vi "edit_component_sequence_dialog.vi"(1 "show configuration?":bool=TRUE, 2 "default folder path":path, 3 "show label?":bool=TRUE, 5 "component specification list in":T1[](array[typedef]), 9 "default":string, 11 "error in (no error)":errorcluster, 12 "choose default?":bool=TRUE, 14 "show settings?":bool=TRUE) -> (6 "component specification list out":T1[](array[typedef]), 10 "default":string, 15 "error out":errorcluster)   [LabVIEW 2010, in "GenericComponent.lvclass"]
uses:
  GenericComponent.lvclass
  clusters/plugin_specification.ctl
  <vilib>/Utility/miscctls.llb/LVPointTypeDef.ctl
panel:
  in  "set_preselected_default":bool=TRUE
  in  "preselected default":string(combo)
  in  "down button":bool
  in  "up button":bool
  in  "cancel button":bool
  in  "edit button":bool
  in  "delete button":bool
  in  "done button":bool
  in  "add button":bool
  in  "Plug-ins":i32(listbox)
  # "Edit component sequence"
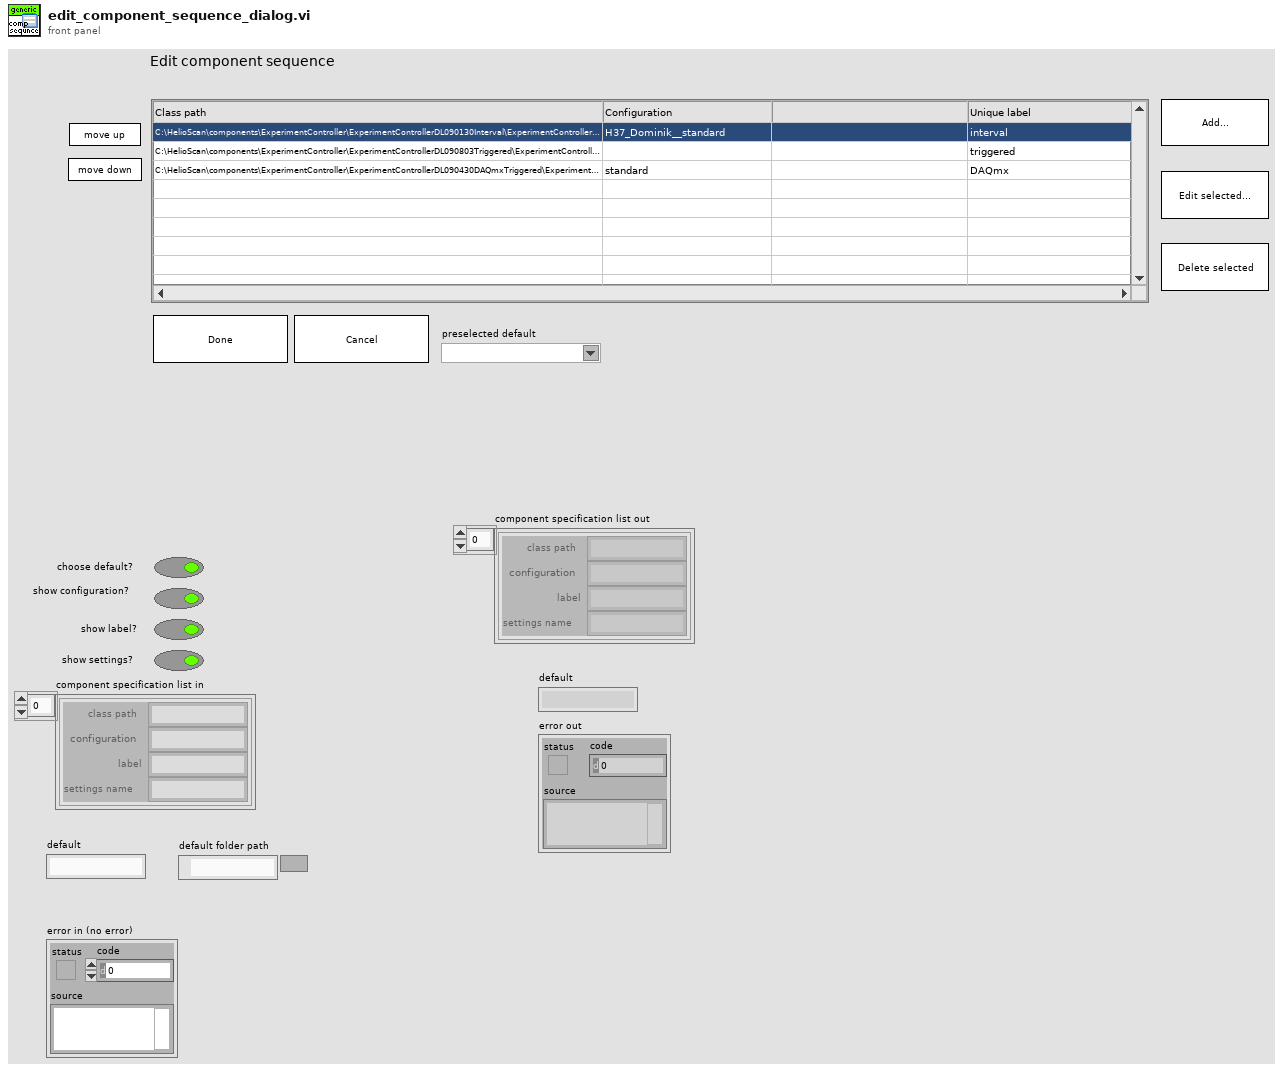
[diagram p1: front panel]
types:
  T1 = typedef "plugin_specification.ctl" = cluster{"class path":string, "configuration":string, "label":string, "settings name":string}
  T2 = typedef "LVPointTypeDef.ctl" = cluster{"Horizontal":i16, "Vertical":i16}
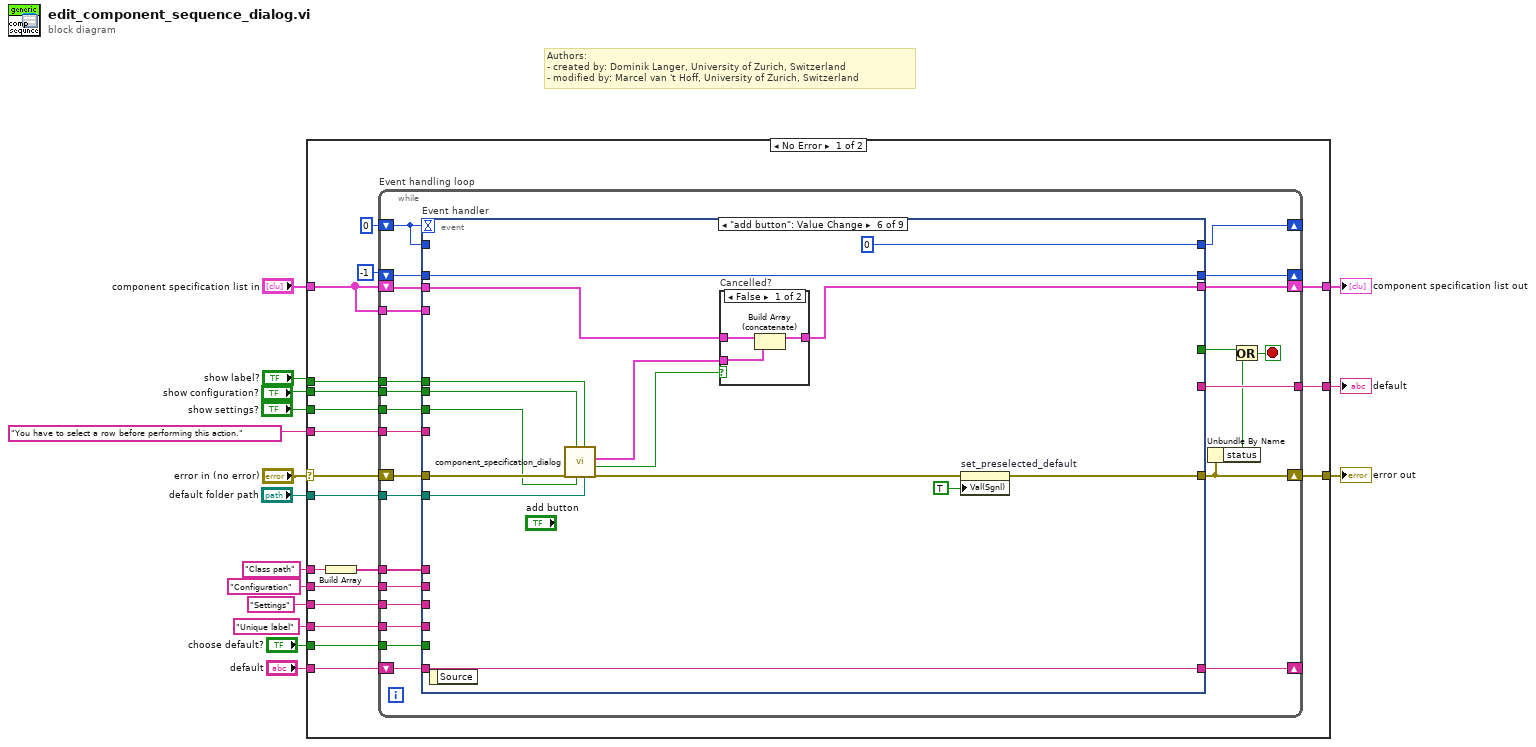
[diagram p0: block diagram]
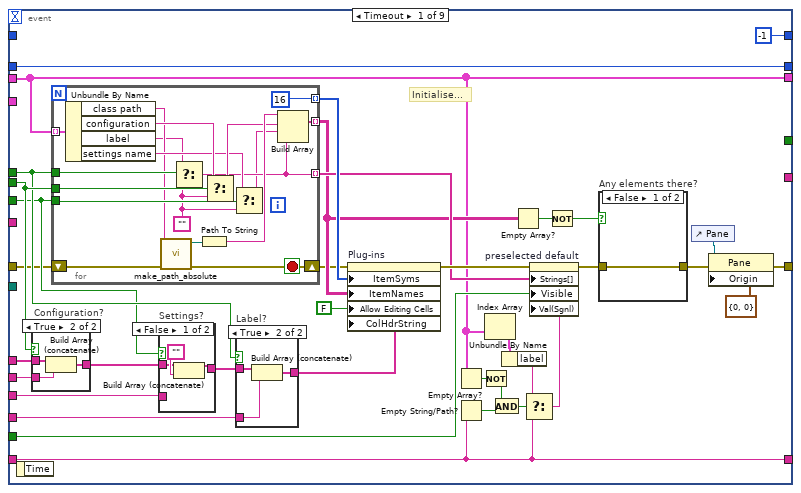
[diagram p2: hidden frame]
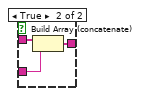
[diagram p3: hidden frame]
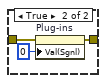
[diagram p4: hidden frame]
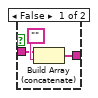
[diagram p5: hidden frame]
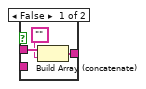
[diagram p6: hidden frame]
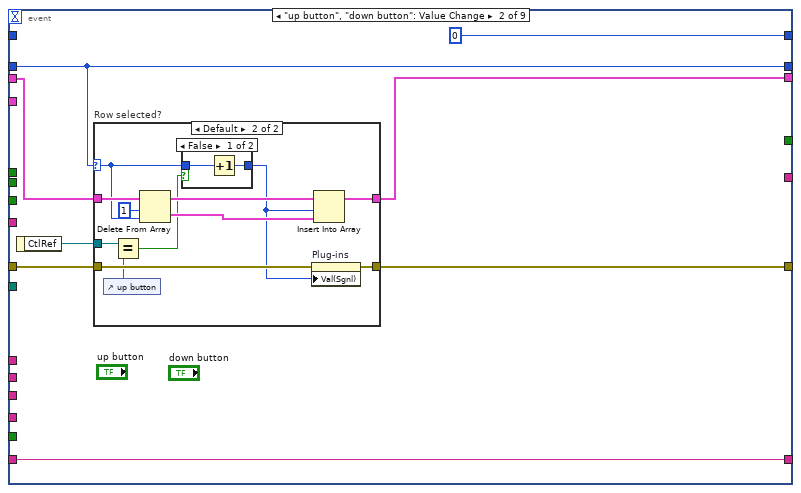
[diagram p7: hidden frame]
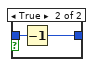
[diagram p9: hidden frame]
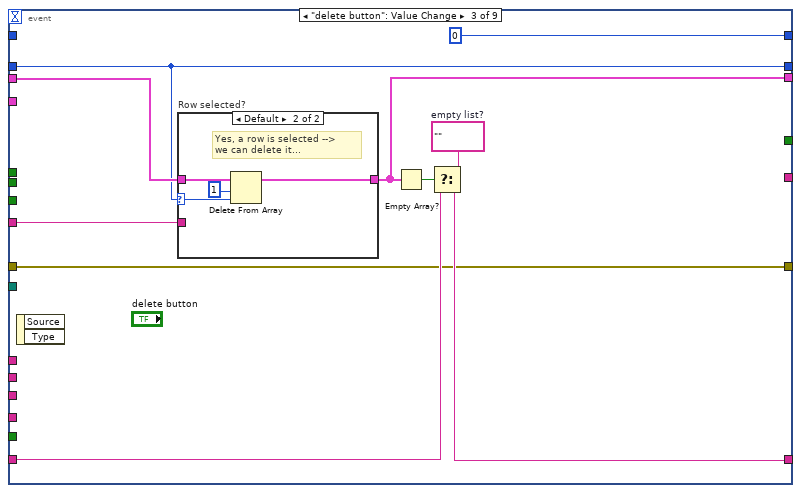
[diagram p10: hidden frame]
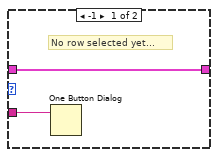
[diagram p11: hidden frame]
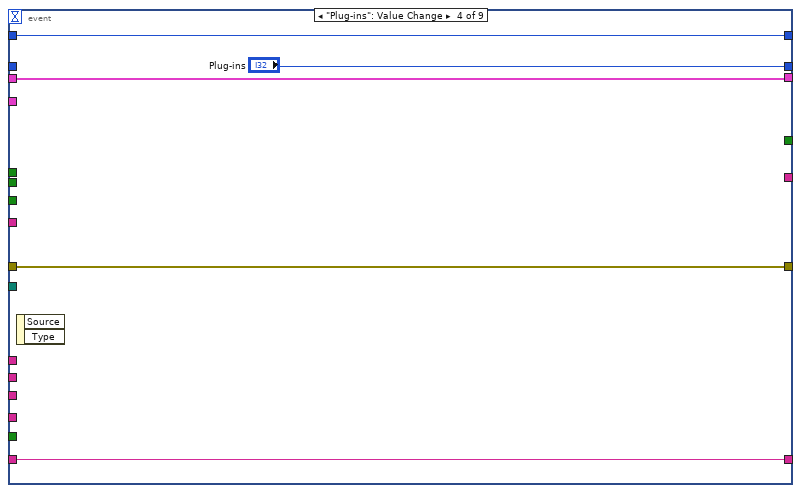
[diagram p12: hidden frame]
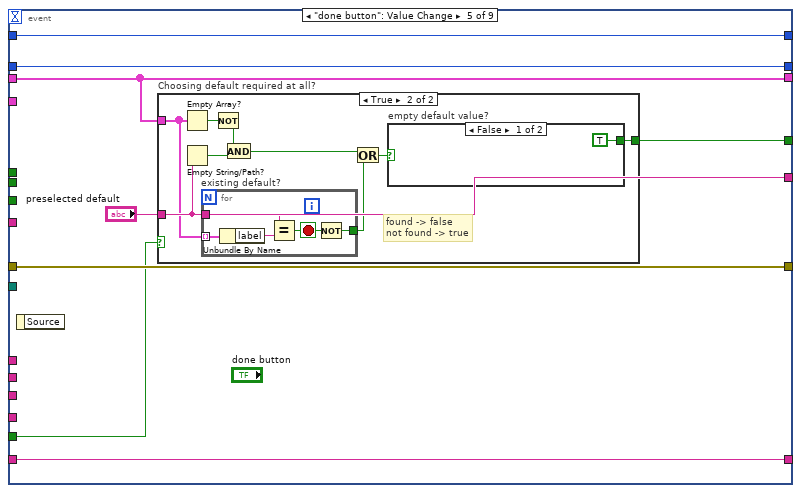
[diagram p13: hidden frame]
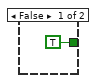
[diagram p14: hidden frame]
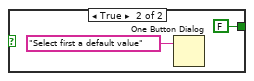
[diagram p15: hidden frame]
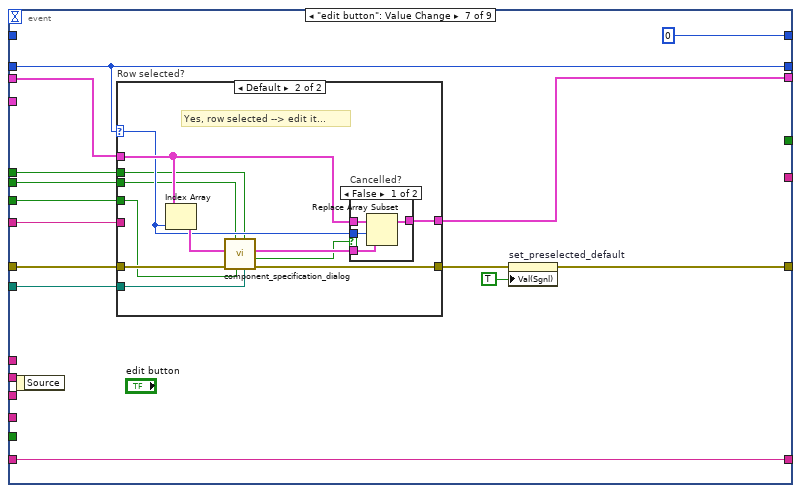
[diagram p17: hidden frame]
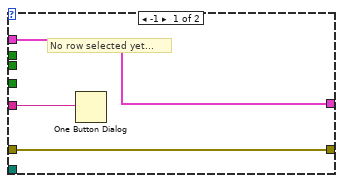
[diagram p18: hidden frame]
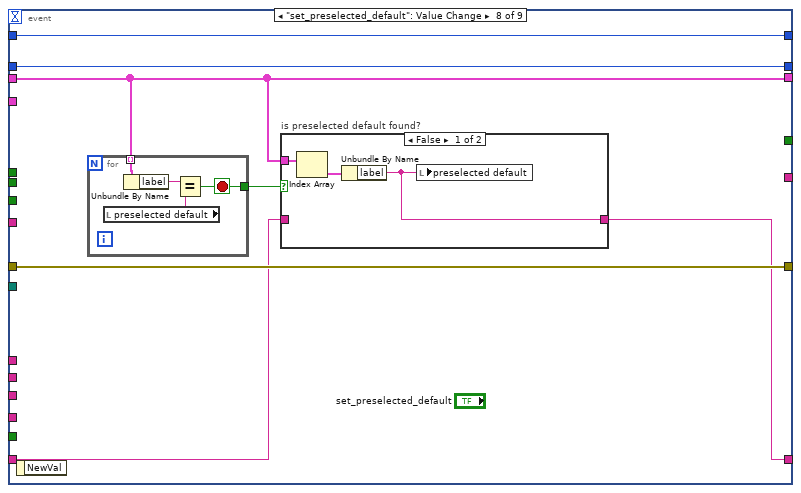
[diagram p20: hidden frame]
diagram:
  # "Authors: \n- created by: Dominik Langer, University of Zurich, Switzerland\n- modified by: Marcel van 't Hoff, University of Zurich, Switzerland"
  n1 = case shown="No Error" "error in (no error)" {
    selector: "error in (no error)" -> [w35 w284]
    tunnel: [w34 w284] -> w15
    tunnel: "component specification list in" -> [w31 _]
    tunnel: "You have to select a row before performing this action." -> [w30 _]
    tunnel: [w29 _] -> w12
    tunnel: "show configuration?" -> [w28 _]
    tunnel: "show label?" -> [w27 _]
    tunnel: "Class path" -> [w26 _]
    tunnel: "Configuration" -> [w23 _]
    tunnel: "Unique label" -> [w24 _]
    tunnel: "choose default?" -> [w22 _]
    tunnel: [w21 _] -> w5
    tunnel: "default" -> [w20 _]
    tunnel: "show settings?" -> [w19 _]
    tunnel: "Settings" -> [w18 _]
    tunnel: "default folder path" -> [w17 _]
    frame No Error {
      n2 = Build Array(w26) -> (w25:string[])
      n3 = while "Event handling loop" {
        shift-right: [w40] -> w34
        shift-left: w35 -> [w60]
        shift-right: [w58] -> _
        shift-left: 0 -> [w59]
        shift-right: [w56] -> w29
        shift-left: w31 -> [w57]
        shift-right: [w54] -> _
        shift-left: -1 -> [w55]
        tunnel: w31 -> [w53]
        tunnel: w30 -> [w52]
        tunnel: w28 -> [w51]
        tunnel: w27 -> [w50]
        tunnel: w25 -> [w49]
        tunnel: w23 -> [w48]
        tunnel: w24 -> [w47]
        tunnel: w22 -> [w46]
        tunnel: [w45] -> w21
        tunnel: w19 -> [w43]
        tunnel: w18 -> [w42]
        tunnel: w17 -> [w41]
        shift-right: [w36] -> _
        shift-left: w20 -> [w44]
        stop <- w37 stop-if-true
        n4 = event "Event handler" shown="[5] \"add button\": Value Change" {
          selector: _ -> [_ _ _ _ _ _ _ _ _]
          dyn-events: _ -> [_ _ _ _ _ _ _ _ _]
          timeout: w59 -> [_ _ _ _ _ _ _ _ _]
          tunnel: w60 -> [w75 w141 w163 w182 w190 w224 w242 w267 w282]
          tunnel: w59 -> [_ _ _ w183 w191 _ _ w269 w283]
          tunnel: [-1 0 0 w183 w191 0 0 w269 w283] -> w58
          tunnel: [w63 w140 w163 w182 w190 w212 w230 w267 w282] -> w40
          tunnel: w57 -> [w69 w143 w172 w181 w187 w219 w241 w264 _]
          tunnel: [_ _ _ _ w185 _ _ _ TRUE] -> w38
          tunnel: [w69 w142 w168 w181 w187 w222 w240 w264 w279] -> w56
          tunnel: w55 -> [w93 w139 w170 _ w189 w220 w238 w268 w281]
          tunnel: [w93 w139 w170 "Plug-ins" w189 w220 w238 w268 w281] -> w54
          tunnel: w53 -> [_ _ _ _ _ _ _ _ w279]
          tunnel: w52 -> [_ _ w169 _ _ _ w237 _ _]
          tunnel: w51 -> [w90 _ _ _ _ w216 w236 _ _]
          tunnel: w50 -> [w89 _ _ _ _ w217 w235 _ _]
          tunnel: w49 -> [w92 _ _ _ _ _ _ _ _]
          tunnel: w48 -> [w91 _ _ _ _ _ _ _ _]
          tunnel: w47 -> [w78 _ _ _ _ _ _ _ _]
          tunnel: w46 -> [w86 _ _ _ w184 _ _ _ _]
          tunnel: [_ _ _ _ "preselected default" _ _ _ w278] -> w45
          tunnel: w44 -> [w61 w137 w165 w179 w188 w210 w229 w266 w278]
          tunnel: w43 -> [w76 _ _ _ _ w215 w234 _ _]
          tunnel: w42 -> [w79 _ _ _ _ _ _ _ _]
          tunnel: w41 -> [_ _ _ _ _ w214 w233 _ _]
          tunnel: [w61 w137 w164 w179 w188 w210 w229 w265 w278] -> w36
          event Timeout {
            # "Initialise..."
            n5 = event-data() -> ()  [unwired: 2 out]
            n6 = case "Configuration?" shown="True" w90 {
              tunnel: w92 -> [w115 w118]
              tunnel: w91 -> [_ w117]
              tunnel: [w114 w116] -> w81
              frame False {
                n7 = Build Array (concatenate)(w115, "") -> (w114:string[])
              }
              frame True {
                n8 = Build Array (concatenate)(w118, w117) -> (w116:string[])
              }
            }
            n9 = for {
              tunnel: w69 -> [w136] mode=indexing
              tunnel: [w134] -> w82 mode=indexing
              tunnel: [16] -> w94 mode=indexing
              tunnel: w89 -> [w132]
              tunnel: w90 -> [w131]
              tunnel: [w125] -> w87 mode=indexing
              tunnel: w76 -> [w128]
              shift-right: [w119] -> w74
              shift-left: w75 -> [w123]
              stop <- w119 stop-if-true
              w126 = ""
              n10 = Unbundle By Name(w136) -> ("class path"=w122:string, "configuration"=w130:string, "label"=w120:string, "settings name"=w127:string)
              n11 = call "make_path_absolute.vi"("error in (no error)"=w123, "relative path"=w122) -> ("error out"=w119:errorcluster, "absolute path"=w121:path)  [unwired: 8 in]
              n12 = Select(t=w120, s=w132, f=w126) -> (s? t:f=w125:string)
              n13 = Path To String(path=w121) -> (string=w135:string)
              n14 = Select(t=w130, s=w131, f=w126) -> (s? t:f=w129:string)
              n15 = Select(t=w127, s=w128, f=w126) -> (s? t:f=w124:string)
              n16 = Build Array(w135, w129, w124, w125) -> (w134:string[])
            }
            n17 = case "Settings?" shown="False" w76 {
              tunnel: w81 -> [w98 w102]
              tunnel: w79 -> [_ w101]
              tunnel: [w97 w100] -> w80
              frame False {
                n18 = Build Array (concatenate)(w98, "") -> (w97:string[])
              }
              frame True {
                n19 = Build Array (concatenate)(w102, w101) -> (w100:string[])
              }
            }
            n20 = case "Label?" shown="True" w89 {
              tunnel: w80 -> [w107 w112]
              tunnel: w78 -> [_ w111]
              tunnel: [w108 w110] -> w77
              frame False {
                n21 = Build Array (concatenate)(w107, "") -> (w108:string[])
              }
              frame True {
                n22 = Build Array (concatenate)(w112, w111) -> (w110:string[])
              }
            }
            n23 = property on="Plug-ins" class="MCListbox (strict)"(error in=w74, "ItemSyms"=w94, "ItemNames"=w82, "Allow Editing Cells"=FALSE, "ColHdrString"=w77) -> (error out=w88:errorcluster)  [unwired: 1 in, 1 out]
            n24 = Empty Array?(array=w69) -> (empty?=w73:bool)
            n25 = Empty String/Path?(string/path=w61) -> (empty?=w71:bool)
            n26 = Not(x=w73) -> (.not. x?=w72:bool)
            n27 = Index Array(array=w69) -> (element=w70:T1)  [unwired: 1 in]
            n28 = And(x=w72, y=w71) -> (x .and. y?=w67:bool)
            n29 = Unbundle By Name(w70) -> ("label"=w68:string)
            n30 = Empty Array?(array=w82) -> (empty?=w84:bool)
            n31 = Select(t=w68, s=w67, f=w61) -> (s? t:f=w66:string)
            n32 = property on="preselected default" class="CmbBox"(error in=w88, "Strings[]"=w87, "Visible"=w86, "Val(Sgnl)"=w66) -> (error out=w85:errorcluster)  [unwired: 1 in, 1 out]
            n33 = Not(x=w84) -> (.not. x?=w83:bool)
            n34 = case "Any elements there?" shown="False" w83 {
              tunnel: w85 -> [w103 w106]
              tunnel: [w103 w105] -> w62
              frame False {
              }
              frame True {
                n35 = property on="Plug-ins" class="MCListbox (strict)"(error in=w106, "Val(Sgnl)"=0 ("Value (Signaling)")) -> (error out=w105:errorcluster)  [unwired: 1 in, 1 out]
              }
            }
            n36 = control-ref of="Pane"() -> (w64:refnum<vi>)
            n37 = property class="Pane"(reference=w64, error in=w62, "Origin"=T2 {"Horizontal"=0, "Vertical"=0}) -> (error out=w63:errorcluster)  [unwired: 1 out]
          }
          event "up button", "down button": Value Change {
            n38 = event-data() -> ("CtlRef"=w138:refnum<vi>)  [unwired: 1 out]
            n39 = case "Row selected?" shown="Default" w139 {
              selector: w139 -> [_ w153]
              tunnel: w143 -> [w146 w155]
              tunnel: [w146 w154] -> w142
              tunnel: w141 -> [w145 w152]
              tunnel: [w145 w151] -> w140
              tunnel: w138 -> [_ w149]
              frame -1 {
              }
              frame Default {
                n40 = control-ref of="up button"() -> (w148:refnum<vi>)
                n41 = Equal?(x=w149, y=w148) -> (x = y?=w147:bool)
                n42 = Delete From Array(array=w155, length=1, index=w153) -> (deleted portion=w156:T1[], array with subset deleted=w157:T1[])
                n43 = case shown="False" w147 {
                  tunnel: w153 -> [w160 w162]
                  tunnel: [w159 w161] -> w150
                  frame False {
                    n44 = Increment(x=w160) -> (x+1=w159:i32)
                  }
                  frame True {
                    n45 = Decrement(x=w162) -> (x-1=w161:i32)
                  }
                }
                n46 = property on="Plug-ins" class="MCListbox (strict)"(error in=w152, "Val(Sgnl)"=w150) -> (error out=w151:errorcluster)  [unwired: 1 in, 1 out]
                n47 = Insert Into Array(array=w157, index=w150, new element=w156) -> (w154:T1[])
              }
            }
          }
          event "delete button": Value Change {
            w167 = ""  # empty list?
            n48 = event-data() -> ()  [unwired: 3 out]
            n49 = case "Row selected?" shown="Default" w170 {
              selector: w170 -> [_ w175]
              tunnel: w172 -> [w173 w178]
              tunnel: [w173 w177] -> w168
              tunnel: w169 -> [w174 _]
              frame -1 {
                # "No row selected yet..."
                n50 = One Button Dialog(message=w174) -> ()  [unwired: 2 out]
              }
              frame Default {
                # "Yes, a row is selected --> \nwe can delete it..."
                n51 = Delete From Array(array=w178, length=1, index=w175) -> (array with subset deleted=w177:T1[])  [unwired: 1 out]
              }
            }
            n52 = Empty Array?(array=w168) -> (empty?=w166:bool)
            n53 = Select(t=w167, s=w166, f=w165) -> (s? t:f=w164:string)
          }
          event "Plug-ins": Value Change {
            n54 = event-data() -> ()  [unwired: 3 out]
          }
          event "done button": Value Change {
            n55 = event-data() -> ()  [unwired: 2 out]
            n56 = case "Choosing default required at all?" shown="True" w184 {
              tunnel: w187 -> [_ w198]
              tunnel: "preselected default" -> [_ w197]
              tunnel: [TRUE w196] -> w185
              frame False {
              }
              frame True {
                # "found -> false\nnot found -> true"
                n57 = Empty Array?(array=w198) -> (empty?=w201:bool)
                n58 = Empty String/Path?(string/path=w197) -> (empty?=w199:bool)
                n59 = for "existing default?" {
                  tunnel: w198 -> [w206] mode=indexing
                  tunnel: w197 -> [w204]
                  tunnel: [w202] -> w195
                  stop <- w203 stop-if-true
                  n60 = Unbundle By Name(w206) -> ("label"=w205:string)
                  n61 = Equal?(x=w204, y=w205) -> (x = y?=w203:bool)
                  n62 = Not(x=w203) -> (.not. x?=w202:bool)
                }
                n63 = Not(x=w201) -> (.not. x?=w200:bool)
                n64 = And(x=w200, y=w199) -> (x .and. y?=w194:bool)
                n65 = Or(x=w194, y=w195) -> (x .or. y?=w193:bool)
                n66 = case "empty default value?" shown="False" w193 {
                  tunnel: [TRUE FALSE] -> w196
                  frame False {
                  }
                  frame True {
                    n67 = One Button Dialog(message="Select first a default value") -> ()  [unwired: 1 in, 1 out]
                  }
                }
              }
            }
          }
          event "add button": Value Change {
            n68 = event-data() -> ()  [unwired: 2 out]
            n69 = call "component_specification_dialog.vi"("default folder path"=w214, "show label?"=w217, "show settings?"=w215, "show configuration?"=w216, "error in (no error)"=w224) -> ("error out"=w213:errorcluster, "cancelled?"=w218:bool, "component specification out"=w223:T1)  [unwired: 4 in]
            n70 = case "Cancelled?" shown="False" w218 {
              tunnel: w223 -> [w227 _]
              tunnel: [w226 w228] -> w222
              tunnel: w219 -> [w225 w228]
              frame False {
                n71 = Build Array (concatenate)(w225, w227) -> (w226:T1[])
              }
              frame True {
              }
            }
            n72 = property on="set_preselected_default" class="Bool (strict)"(error in=w213, "Val(Sgnl)"=TRUE ("Value (Signaling)")) -> (error out=w212:errorcluster)  [unwired: 1 in, 1 out]
          }
          event "edit button": Value Change {
            n73 = event-data() -> ()  [unwired: 2 out]
            n74 = case "Row selected?" shown="Default" w238 {
              selector: w238 -> [_ w251]
              tunnel: w242 -> [w245 w257]
              tunnel: [w245 w256] -> w231
              tunnel: w241 -> [w244 w254]
              tunnel: [w244 w253] -> w240
              tunnel: w237 -> [w243 _]
              tunnel: w236 -> [_ w249]
              tunnel: w235 -> [_ w248]
              tunnel: w234 -> [_ w247]
              tunnel: w233 -> [_ w246]
              frame -1 {
                # "No row selected yet..."
                n75 = One Button Dialog(message=w243) -> ()  [unwired: 2 out]
              }
              frame Default {
                # "Yes, row selected --> edit it..."
                n76 = Index Array(array=w254, index=w251) -> (element=w255:T1)
                n77 = call "component_specification_dialog.vi"("default folder path"=w246, "show label?"=w248, "show settings?"=w247, "show configuration?"=w249, "error in (no error)"=w257, "component specification in"=w255) -> ("error out"=w256:errorcluster, "cancelled?"=w250:bool, "component specification out"=w252:T1)  [unwired: 3 in]
                n78 = case "Cancelled?" shown="False" w250 {
                  tunnel: w254 -> [w261 w262]
                  tunnel: [w260 w262] -> w253
                  tunnel: w252 -> [w259 _]
                  tunnel: w251 -> [w258 _]
                  frame False {
                    n79 = Replace Array Subset(array=w261, new element=w259, index=w258) -> (w260:T1[])
                  }
                  frame True {
                  }
                }
              }
            }
            n80 = property on="set_preselected_default" class="Bool (strict)"(error in=w231, "Val(Sgnl)"=TRUE ("Value (Signaling)")) -> (error out=w230:errorcluster)  [unwired: 1 in, 1 out]
          }
          event "set_preselected_default": Value Change {
            n81 = event-data() -> ()  [unwired: 2 out]
            n82 = for {
              tunnel: w264 -> [w272] mode=indexing
              tunnel: [w270] -> w263
              stop <- w270 stop-if-true
              n83 = local read "preselected default"() -> (w273:string)
              n84 = Unbundle By Name(w272) -> ("label"=w271:string)
              n85 = Equal?(x=w271, y=w273) -> (x = y?=w270:bool)
            }
            n86 = case "is preselected default found?" shown="False" w263 {
              tunnel: w264 -> [w276 _]
              tunnel: [w274 w277] -> w265
              tunnel: w266 -> [_ w277]
              frame False {
                n87 = Index Array(array=w276) -> (element=w275:T1)  [unwired: 1 in]
                n88 = Unbundle By Name(w275) -> ("label"=w274:string)
                n89 = local write "preselected default"(w274) -> ()
              }
              frame True {
              }
            }
          }
          event "cancel button": Value Change; Panel Close {
            n90 = event-data() -> ()  [unwired: 4 out]
          }
        }
        n91 = Unbundle By Name(w40) -> ("status"=w39:bool)
        n92 = Or(x=w38, y=w39) -> (x .or. y?=w37:bool)
      }
    }
    frame Error {
    }
  }
  "error out" <- w15
  "component specification list out" <- w12
  "default" <- w5
